vi "HTML header.vi"(11 "Title":string) -> (3 "HTML header":string)   [LabVIEW 2012]
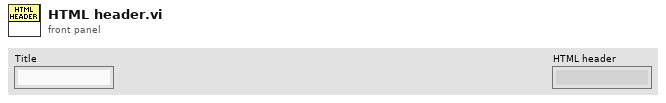
[diagram p1: front panel]
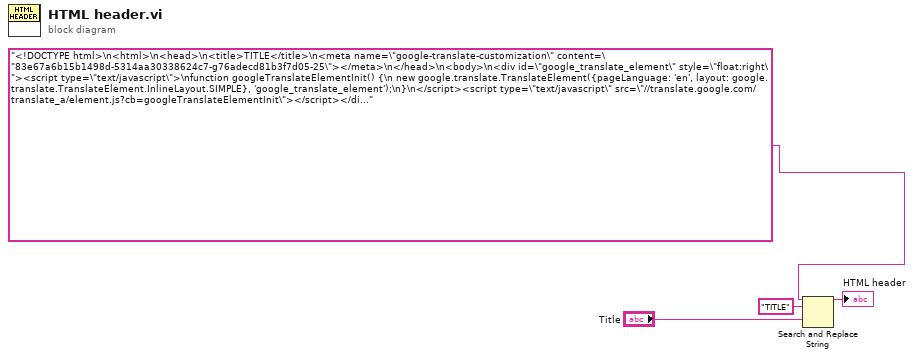
[diagram p0: block diagram]
diagram:
  n1 = Search and Replace String(input string="<!DOCTYPE html>\n<html>\n<head>\n<title>TITLE</title>\n<meta name=\"google-translate-customization\" content=\"83e67a6b15b1498d-5314aa30338624c7-g76adecd81b3f7d05-25\"></meta>\n</head>\n<body>\n<div id=\"google_translate_element\" style=\"float:right\"><script type=\"text/javascript\">\nfunction googleTranslateElementInit() {\n new google.translate.TranslateElement({pageLanguage: 'en', layout: google.translate.TranslateElement.InlineLayout.SIMPLE}, 'google_translate_element');\n}\n</script><script type=\"text/javascript\" src=\"//translate.google.com/translate_a/element.js?cb=googleTranslateElementInit\"></script></div>\n        ", search string="TITLE", replace string="Title") -> (result string=→"HTML header":string)  [unwired: 5 in, 3 out]
